vi "extractADCSubstring.vi"(8 "error in (no error)":errorcluster, 9 "lastIsTrue?":bool, 11 "Model in":refnum<class "Model.lvclass">) -> (0 "error out":errorcluster, 2 "adcElement":i32, 3 "Model out":refnum<class "Model.lvclass">)   [LabVIEW 2013, in "Model.lvclass"]
uses:
  Model.lvclass
  <userlib>/Common/ILC/ILCModelTypedefs/FinalDelimiter.ctl
  Model.lvclass/Model.ctl
  <userlib>/Common/ILC/ILCModelTypedefs/ILCModelTypedefs.lvlib
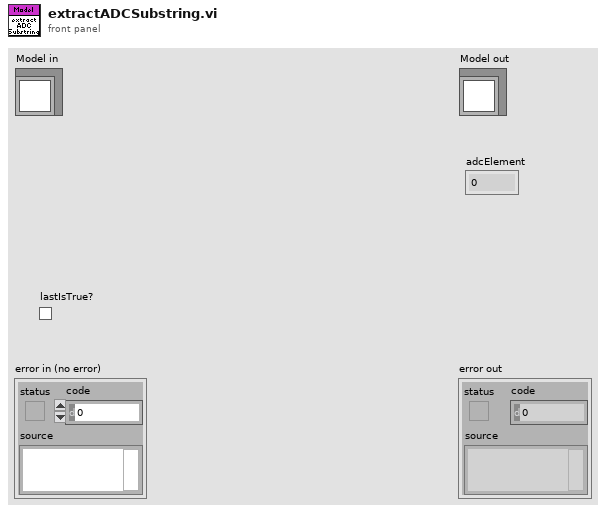
[diagram p1: front panel]
types:
  T1 = typedef "ILCCommon.lvlib/ILCModelTypedefs.lvlib/FinalDelimiter.ctl" = enum16{",", "<CR><LF>"}
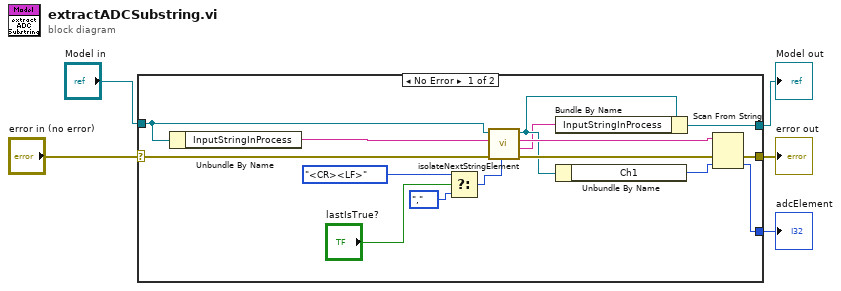
[diagram p0: block diagram]
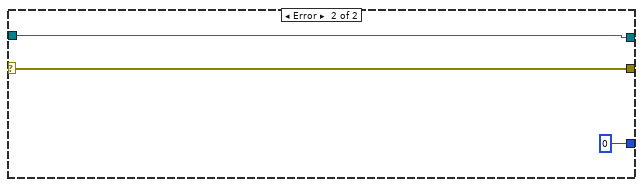
[diagram p2: hidden frame]
diagram:
  n1 = case shown="No Error" "error in (no error)" {
    selector: "error in (no error)" -> [w16 w23]
    tunnel: [w15 w23] -> w4
    tunnel: [w17 w22] -> w2
    tunnel: "Model in" -> [w13 w22]
    tunnel: [w10 0 ("Ch1")] -> w1
    frame No Error {
      n2 = Unbundle By Name(w13) -> ("InputStringInProcess"=w14:string)
      n3 = Select(t=FinalDelimiter."<CR><LF>", s="lastIsTrue?", f=FinalDelimiter."," ("Final Delimiter")) -> (s? t:f=w6:T1)
      n4 = call "isolateNextStringElement.vi"("Final Delimiter"=w6, "error in (no error)"=w16, "inputString"=w14, "Model in"=w13) -> ("error out"=w19:errorcluster, "remainingString"=w11:string, "extractedSegment"=w20:string, "Model out"=w12:refnum<class "Model.lvclass">)  [unwired: 4 in]
      n5 = Bundle By Name(cluster=w12, "InputStringInProcess"=w11) -> (w17:refnum<class "Model.lvclass">)
      n6 = Unbundle By Name(w12) -> ("Ch1"=w18:i32)
      n7 = Scan From String(input string=w20, error in=w19, default 1=w18) -> (error out=w15:errorcluster, output 1=w10:i32)  [unwired: 2 in, 2 out]
    }
    frame Error {
    }
  }
  "error out" <- w4
  "Model out" <- w2
  "adcElement" <- w1
